vi "connect.vi"(8 "error in (no error)":errorcluster, 10 "VISA resource name":refnum<visa-resource-name>, 11 "RS in":refnum<class "RS.lvclass">) -> (0 "error out":errorcluster, 2 "VISA resource name out":refnum<visa-resource-name>, 3 "RS out":refnum<class "RS.lvclass">)   [LabVIEW 2015, in "RS.lvclass"]
uses:
  RS.lvclass
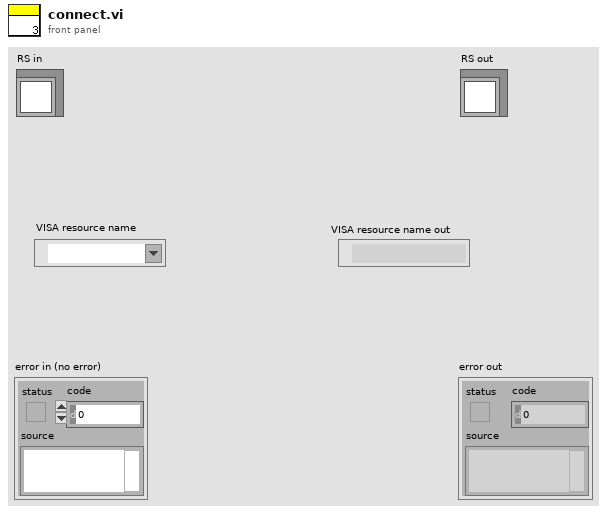
[diagram p1: front panel]
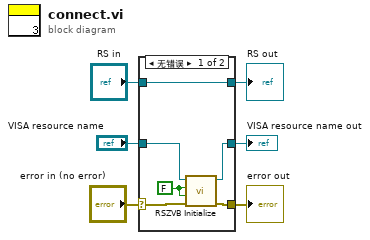
[diagram p0: block diagram]
diagram:
  n1 = case shown="无错误" "error in (no error)" {
    selector: "error in (no error)" -> [w9 w15]
    tunnel: [w8 w15] -> w5
    tunnel: [w12 w14] -> w3
    tunnel: "RS in" -> [w12 w14]
    tunnel: "VISA resource name" -> [w11 w13]
    tunnel: [w7 w13] -> w1
    frame No Error {
      w10 = FALSE ("Reset? (T: Yes)")
      n2 = call "RSZVB Initialize.vi"("error in (no error)"=w9, "Reset? (T: Yes)"=w10, "ID Query? (T: Yes)"=w10, "VISA Resource Name (GPIB::20)"=w11) -> ("error out"=w8:errorcluster, "dup VISA session"=w7:refnum<visa-resource-name>)  [unwired: 6 in]
    }
    frame Error {
    }
  }
  "error out" <- w5
  "RS out" <- w3
  "VISA resource name out" <- w1
